vi "Generate Error Handling DVR.vi"(8 "Error In":errorcluster, 11 "Error Handling In":refnum<class "Error Handling.lvclass">) -> (0 "Error Out":errorcluster, 3 "Error Handling Out":refnum<class "Error Handling.lvclass">)   [LabVIEW 2021, in "Error Handling.lvclass"]
uses:
  Error Handling.lvclass
  Controls/Data.ctl
  Error Handling.lvclass/Error Handling.ctl
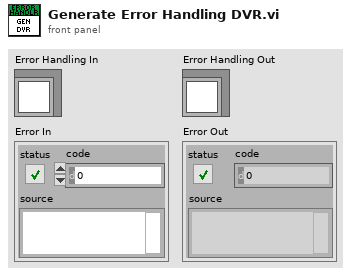
[diagram p1: front panel]
types:
  T1 = typedef "Error Handling.lvclass/Data.ctl" = cluster{"Log File Reference":refnum<file>}
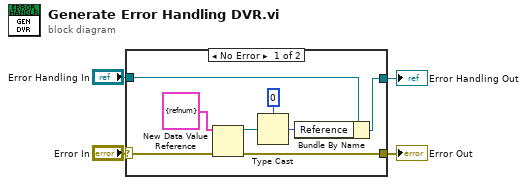
[diagram p0: block diagram]
diagram:
  n1 = case shown="No Error" "Error In" {
    selector: "Error In" -> [w12 w14]
    tunnel: "Error Handling In" -> [w9 w13]
    tunnel: [w8 w13] -> w3
    tunnel: [w7 w14] -> w1
    frame No Error {
      n2 = New Data Value Reference(data value=T1 {"Log File Reference"=refnum} ("Data"), error in=w12) -> (data value reference=w11:refnum<data-value>, error out=w7:errorcluster)
      n3 = Type Cast(type=u64 0, x=w11) -> (*(type *) &x=w6:u64)
      n4 = Bundle By Name(cluster=w9, "Reference"=w6) -> (w8:refnum<class "Error Handling.lvclass">)
    }
    frame Error {
    }
  }
  "Error Out" <- w1
  "Error Handling Out" <- w3
